vi "configFile to XML.vi"(1 "configuration file path":path) -> (0 "output cluster":T2 {"Image Settings"."2nd Axis" items=["x", "y", "z"]; "Image Settings"."1st Axis" items=["x", "y", "z"]; "Image Settings"."Time Resolution\n(ms/pixel)" format="%.2f"; "Image Settings"."Image Resolution (nm/pixel)"."z" format="%.2f"; "Image Settings"."Image Resolution (nm/pixel)"."y" format="%.2f"; "Image Settings"."Image Resolution (nm/pixel)"."x" format="%.2f"; "Image Settings"."Image Size (µm)"."z" format="%.2f"; "Image Settings"."Image Size (µm)"."y" format="%.2f"; "Image Settings"."Image Size (µm)"."x" format="%.2f"; "Image Settings"."End Position (µm)"."z" format="%.2f"; "Image Settings"."End Position (µm)"."y" format="%.2f"; "Image Settings"."End Position (µm)"."x" format="%.2f"; "Image Settings"."Start Position (µm)"."z" format="%.2f"; "Image Settings"."Start Position (µm)"."y" format="%.2f"; "Image Settings"."Start Position (µm)"."x" format="%.2f"})   [LabVIEW 2009]
uses:
  ImageSettings.ctt
  <vilib>/Utility/config.llb/Read Key (Double).vi
  <vilib>/Utility/config.llb/NI_LVConfig.lvlib
panel:
  in  "FIFO Settings":T3={"Measurement"={"Binning (ms)"=0.001, "External Trigger Condition"=0, "Stop Condition:"=0, "Stop Count"=0.0, "Buffer Size (Photons)"=30000, "No of Channels"=1, "Ext Latch Delay"=0}, "ADC"={"Module"=0, "ADC Resolution"=0, "Dither Range"=0, "Count Increment"=0, "Macro Time Clock"=0}, "SYNC"={"SYNC ZC Level (mV)"=-49.889763, "SYNC Freq Divider"=1, "SYNC Holdoff (ns)"=4.0, "SYNC Threshold (mV)"=-19.607843}, "TAC"={"TAC Range (ns)"=50.0, "TAC Gain"=1, "TAC Offset (%)"=0.0, "TAC Limit Low (%)"=0.0, "TAC Limit High (%)"=100.0}, "CFD"={"CFD Limit Low (mV)"=-43.137257, "CFD Limit High (mV)"=67.76471, "CFD ZC Level (mV)"=-49.889763, "CFD Holdoff (ns)"=5.0}} {"CFD"."CFD Holdoff (ns)" min=5 max=20 format="%.2f"; "CFD"."CFD ZC Level (mV)" min=-96 max=96 format="%.2f"; "CFD"."CFD Limit High (mV)" min=4 max=80 format="%.2f"; "CFD"."CFD Limit Low (mV)" min=-500 max=80 format="%.2f"; "TAC"."TAC Limit High (%)" min=0 max=100 format="%.2f"; "TAC"."TAC Limit Low (%)" min=0 max=100 format="%.2f"; "TAC"."TAC Offset (%)" min=0 max=100 format="%.2f"; "TAC"."TAC Gain" min=1 max=15 step=1; "TAC"."TAC Range (ns)" min=50 max=2000 format="%.2f"; "SYNC"."SYNC Threshold (mV)" min=-500 max=-19 format="%.2f"; "SYNC"."SYNC Holdoff (ns)" min=4 max=16 format="%.2f"; "SYNC"."SYNC Freq Divider" min=1 max=16 step=1; "SYNC"."SYNC ZC Level (mV)" min=-96 max=96 format="%.2f"; "ADC"."Macro Time Clock" items=["Internal (50ns)", "Sync-Trigger", "1/2 Sync-Trigger"]; "ADC"."Module" items=["SPC 630", "SPC 830", "SPC 13x", "HydraHarp"]; "ADC"."Count Increment" min=1 max=255 step=1; "ADC"."Dither Range" min=0 max=256 step=32; "Measurement"."Ext Latch Delay" min=0 max=255 step=1; "Measurement"."Stop Count" format="%.2f"; "Measurement"."Stop Condition:" items=["None", "Photon Count", "Time (s)"]; "Measurement"."External Trigger Condition" max=2 step=1; "Measurement"."No of Channels" max=14; "Measurement"."Binning (ms)" min=1e-07 max=100000 format="%.3f"}
  out "value":i32
  in  "Image Settings":T1={"Start Position (µm)"={"x"=0.0, "y"=0.0, "z"=0.0}, "End Position (µm)"={"x"=10.0, "y"=10.0, "z"=0.0}, "Image Resolution (nm/pixel)"={"x"=50.0, "y"=50.0, "z"=100.0}, "Image Size (µm)"={"x"=10.0, "y"=10.0, "z"=0.0}, "Image Size (pixel)"={"x"=50, "y"=50, "z"=0}, "Time Resolution\n(ms/pixel)"=7.0, "1st Axis"=0, "2nd Axis"=1, "Retrace"=FALSE, "Estimated Time"=""} {"2nd Axis" items=["x", "y", "z"]; "1st Axis" items=["x", "y", "z"]; "Time Resolution\n(ms/pixel)" format="%.2f"; "Image Resolution (nm/pixel)"."z" format="%.2f"; "Image Resolution (nm/pixel)"."y" format="%.2f"; "Image Resolution (nm/pixel)"."x" format="%.2f"; "Image Size (µm)"."z" format="%.2f"; "Image Size (µm)"."y" format="%.2f"; "Image Size (µm)"."x" format="%.2f"; "End Position (µm)"."z" format="%.2f"; "End Position (µm)"."y" format="%.2f"; "End Position (µm)"."x" format="%.2f"; "Start Position (µm)"."z" format="%.2f"; "Start Position (µm)"."y" format="%.2f"; "Start Position (µm)"."x" format="%.2f"}
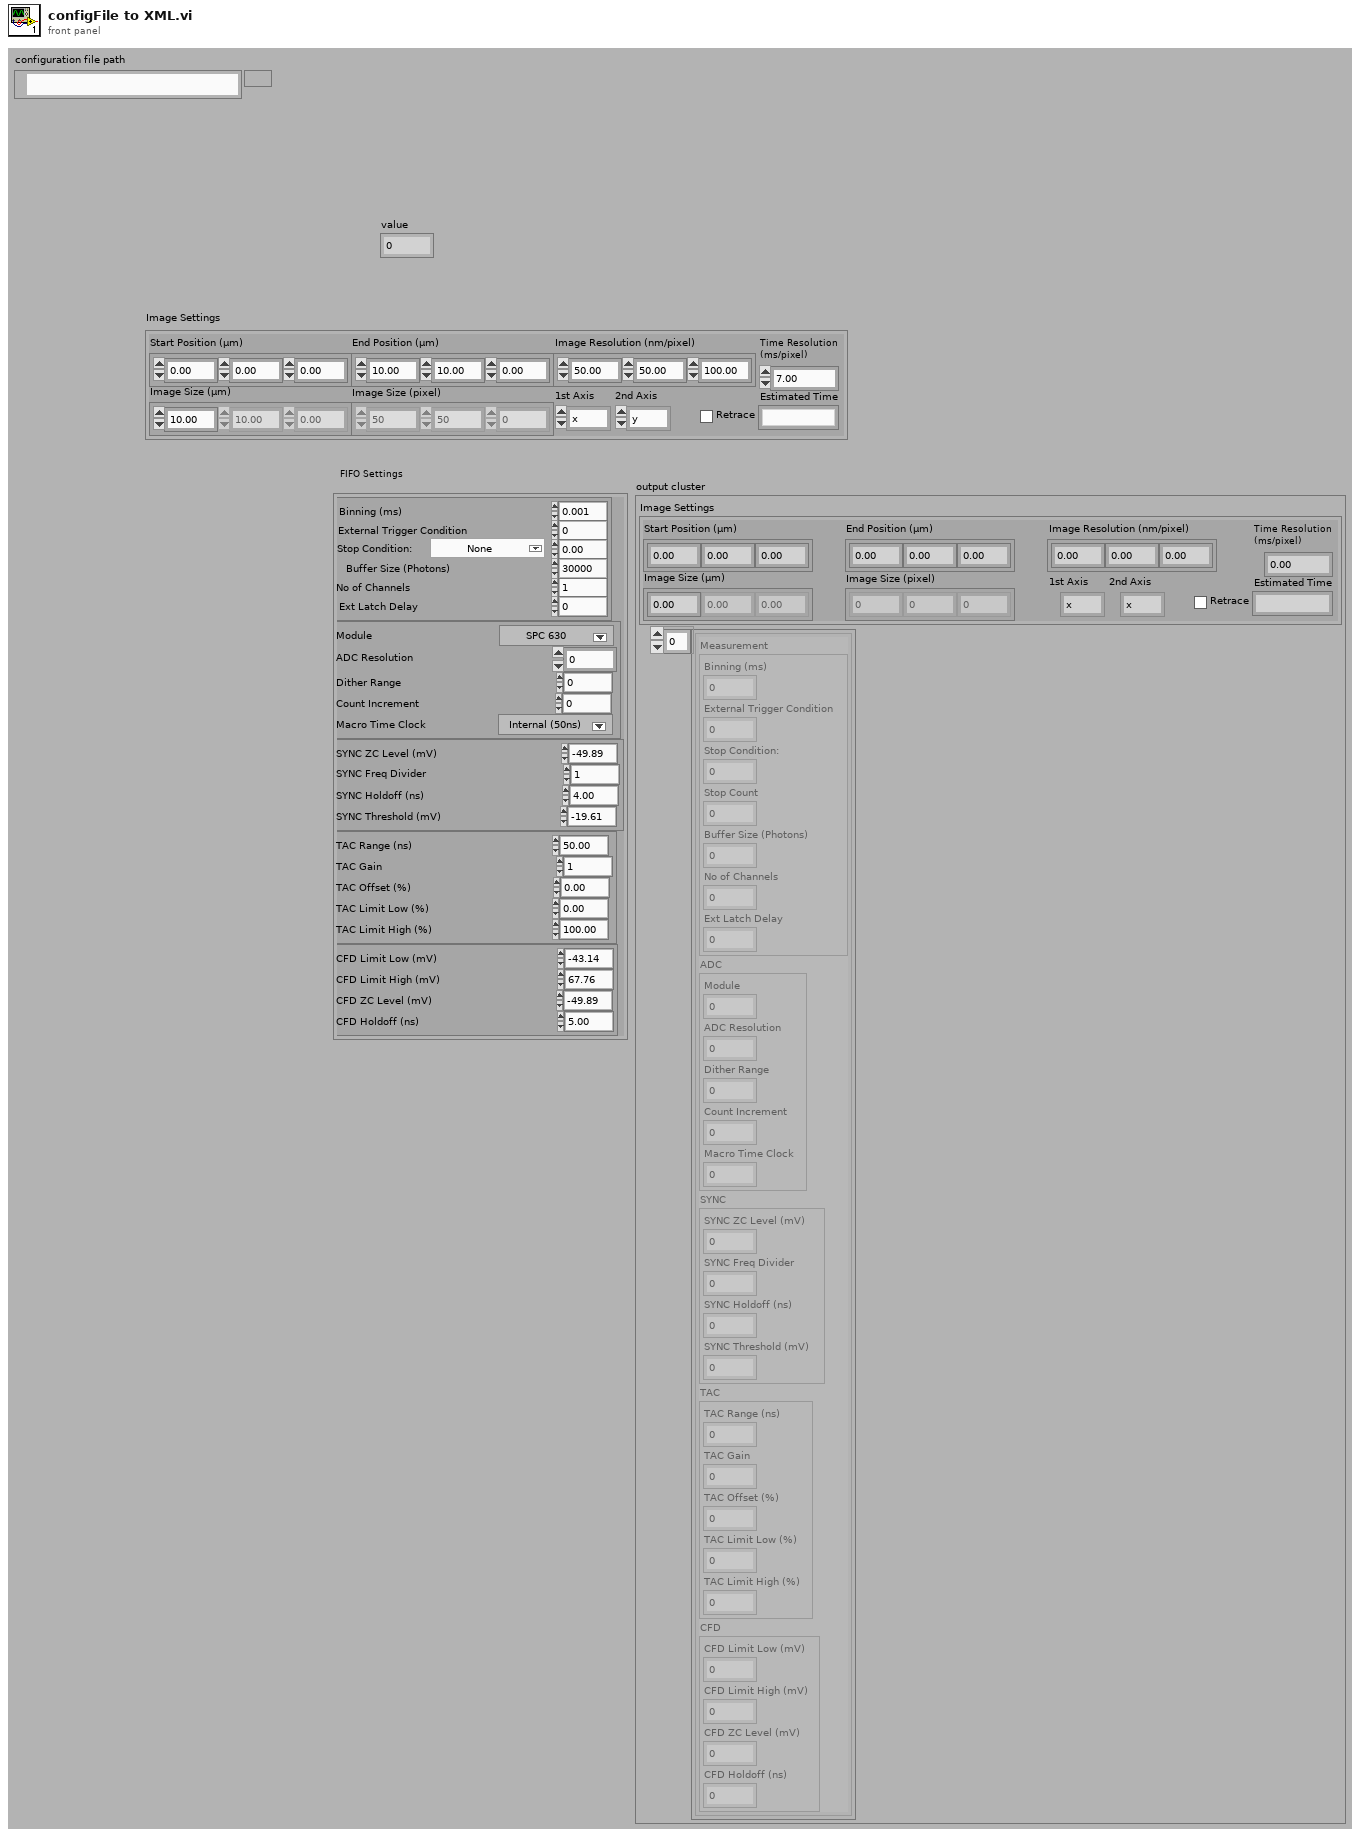
[diagram p1: front panel]
types:
  T1 = typedef "ImageSettings.ctt" = cluster{"Start Position (µm)":cluster{"x":dbl, "y":dbl, "z":dbl}, "End Position (µm)":cluster{"x":dbl, "y":dbl, "z":dbl}, "Image Resolution (nm/pixel)":cluster{"x":dbl, "y":dbl, "z":dbl}, "Image Size (µm)":cluster{"x":dbl, "y":dbl, "z":dbl}, "Image Size (pixel)":cluster{"x":u32, "y":u32, "z":u32}, "Time Resolution\n(ms/pixel)":dbl, "1st Axis":u16, "2nd Axis":u16, "Retrace":bool, "Estimated Time":string}
  T2 = cluster{"Image Settings":T1, cluster{"Measurement":cluster{"Binning (ms)":sgl, "External Trigger Condition":u16, "Stop Condition:":u16, "Stop Count":dbl, "Buffer Size (Photons)":u16, "No of Channels":u16, "Ext Latch Delay":i16}, "ADC":cluster{"Module":u16, "ADC Resolution":i32, "Dither Range":i16, "Count Increment":i16, "Macro Time Clock":i16}, "SYNC":cluster{"SYNC ZC Level (mV)":sgl, "SYNC Freq Divider":i16, "SYNC Holdoff (ns)":sgl, "SYNC Threshold (mV)":sgl}, "TAC":cluster{"TAC Range (ns)":sgl, "TAC Gain":i16, "TAC Offset (%)":sgl, "TAC Limit Low (%)":sgl, "TAC Limit High (%)":sgl}, "CFD":cluster{"CFD Limit Low (mV)":sgl, "CFD Limit High (mV)":sgl, "CFD ZC Level (mV)":sgl, "CFD Holdoff (ns)":sgl}}[]}
  T3 = cluster{"Measurement":cluster{"Binning (ms)":sgl, "External Trigger Condition":u16, "Stop Condition:":u16, "Stop Count":dbl, "Buffer Size (Photons)":u16, "No of Channels":u16, "Ext Latch Delay":i16}, "ADC":cluster{"Module":u16, "ADC Resolution":i32, "Dither Range":i16, "Count Increment":i16, "Macro Time Clock":i16}, "SYNC":cluster{"SYNC ZC Level (mV)":sgl, "SYNC Freq Divider":i16, "SYNC Holdoff (ns)":sgl, "SYNC Threshold (mV)":sgl}, "TAC":cluster{"TAC Range (ns)":sgl, "TAC Gain":i16, "TAC Offset (%)":sgl, "TAC Limit Low (%)":sgl, "TAC Limit High (%)":sgl}, "CFD":cluster{"CFD Limit Low (mV)":sgl, "CFD Limit High (mV)":sgl, "CFD ZC Level (mV)":sgl, "CFD Holdoff (ns)":sgl}}
  T4 = typedef "NI_LVConfig.lvlib/Config Data RefNum.ctl" = refnum<k1>
  T5 = cluster{"Measurement":cluster{"Binning (ms)":sgl, "External Trigger Condition":u16, "Stop Condition:":u16, "Stop Count":dbl, "Buffer Size (Photons)":u16, "No of Channels":u16, "Ext Latch Delay":i16}, "ADC":cluster{"Module":u16, "ADC Resolution":i32, "Dither Range":i16, "Count Increment":i16, "Macro Time Clock":i16}, "SYNC":cluster{"SYNC ZC Level (mV)":sgl, "SYNC Freq Divider":i16, "SYNC Holdoff (ns)":sgl, "SYNC Threshold (mV)":sgl}, "TAC":cluster{"TAC Range (ns)":sgl, "TAC Gain":i16, "TAC Offset (%)":sgl, "TAC Limit Low (%)":sgl, "TAC Limit High (%)":sgl}, "CFD":cluster{"CFD Limit Low (mV)":sgl, "CFD Limit High (mV)":sgl, "CFD ZC Level (mV)":sgl, "CFD Holdoff (ns)":sgl}}[]
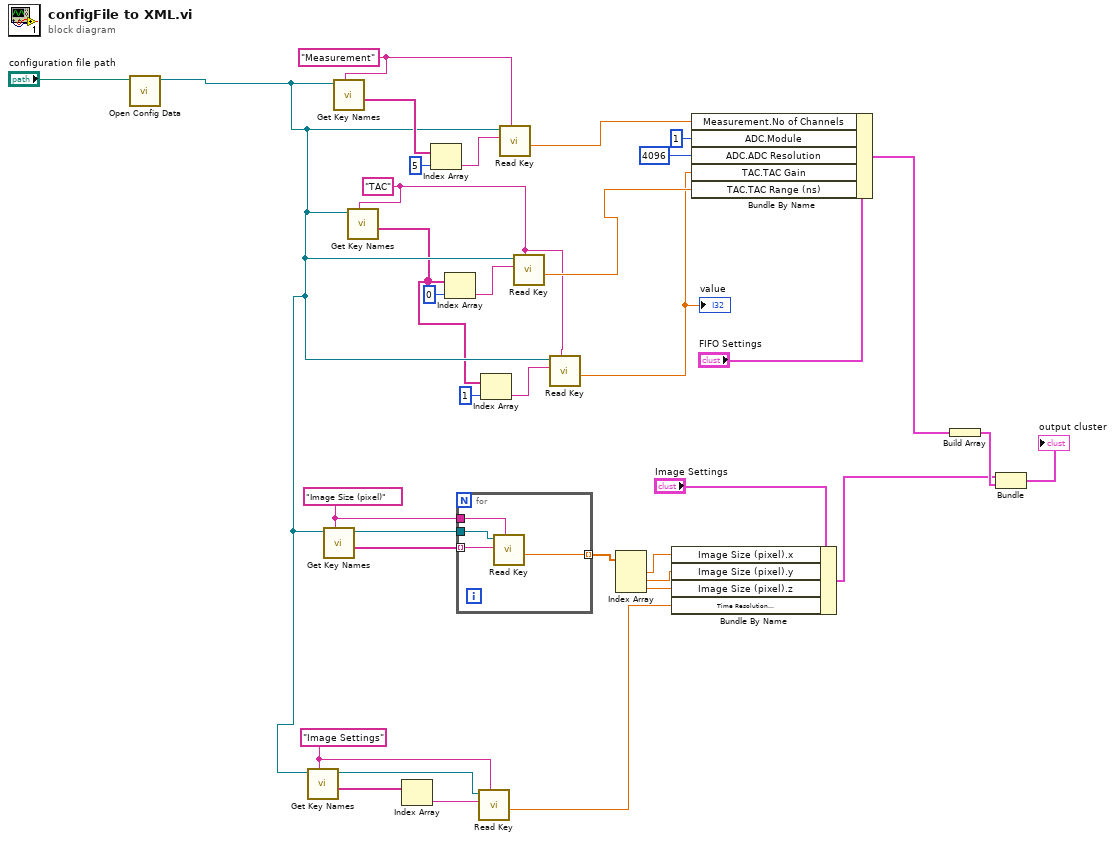
[diagram p0: block diagram]
diagram:
  w5 = "Image Settings" ("section")
  w17 = "Image Size (pixel)" ("section")
  w20 = "TAC" ("section")
  w33 = "Measurement" ("section")
  n1 = call <vilib>:"Open Config Data.vi"("configuration file path"="configuration file path") -> ("refnum"=w11:T4)  [unwired: 8 in, 2 out]
  n2 = call <vilib>:"Get Key Names.vi"("section"=w5, "refnum"=w11) -> ("key names"=w10:string[], "refnum out"=w8:T4)  [unwired: 6 in, 2 out]
  n3 = call <vilib>:"Get Key Names.vi"("section"=w17, "refnum"=w11) -> ("key names"=w19:string[], "refnum out"=w18:T4)  [unwired: 6 in, 2 out]
  n4 = call <vilib>:"Get Key Names.vi"("section"=w33, "refnum"=w11) -> ("key names"=w29:string[])  [unwired: 6 in, 3 out]
  n5 = call <vilib>:"Get Key Names.vi"("section"=w20, "refnum"=w11) -> ("key names"=w1:string[])  [unwired: 6 in, 3 out]
  n6 = Index Array(array=w10) -> (element=w9:string)  [unwired: 1 in]
  n7 = Index Array(array=w29, index=5) -> (element=w32:string)
  n8 = Index Array(array=w1, index=0) -> (element=w28:string)
  n9 = for {
    tunnel: w19 -> [w39] mode=indexing
    tunnel: w18 -> [w38]
    tunnel: w17 -> [w37]
    tunnel: [w36] -> w16 mode=indexing
    n10 = call-poly <vilib>:"Read Key.vi"("section"=w37, "key"=w39, "refnum"=w38) -> ("value"=w36:dbl)  [unwired: 5 in, 3 out]
  }
  n11 = call-poly <vilib>:"Read Key.vi"("section"=w5, "key"=w9, "refnum"=w8) -> ("value"=w7:dbl)  [unwired: 5 in, 3 out]
  n12 = Index Array(array=w1, index=1) -> (element=w23:string)
  n13 = call-poly <vilib>:"Read Key.vi"("section"=w33, "key"=w32, "refnum"=w11) -> ("value"=w30:dbl)  [unwired: 5 in, 3 out]
  n14 = call-poly <vilib>:"Read Key.vi"("section"=w20, "key"=w28, "refnum"=w11) -> ("value"=w24:dbl)  [unwired: 5 in, 3 out]
  n15 = call-poly <vilib>:"Read Key.vi"("section"=w20, "key"=w23, "refnum"=w11) -> ("value"=w21:dbl)  [unwired: 5 in, 3 out]
  "value" <- w21
  n16 = Index Array(array=w16) -> (element #1=w14:dbl, element #2=w13:dbl, element #3=w12:dbl)  [unwired: 3 in]
  n17 = Bundle By Name(cluster="Image Settings", "Image Size (pixel).x"=w14, "Image Size (pixel).y"=w13, "Image Size (pixel).z"=w12, "Time Resolution\n(ms/pixel)"=w7) -> (w6:T1)
  n18 = Bundle By Name(cluster="FIFO Settings", "Measurement.No of Channels"=w30, "ADC.Module"=u16 1, "ADC.ADC Resolution"=4096, "TAC.TAC Gain"=w21, "TAC.TAC Range (ns)"=w24) -> (w4:T3)
  n19 = Build Array(w4) -> (w34:T5)
  n20 = Bundle("Image Settings"=w6, w34) -> (→"output cluster":T2)  [unwired: 1 in]
